vi "AsynCall - MBus Handler.vi"(8 "error in (no error)":errorcluster) -> (0 "error out":errorcluster)   [LabVIEW 2018]
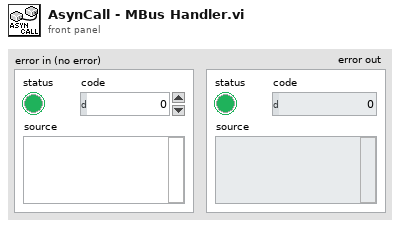
[diagram p1: front panel]
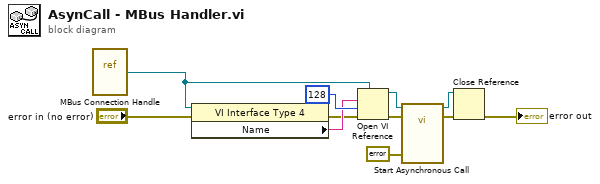
[diagram p0: block diagram]
diagram:
  n1 = vi-ref "MBus Connection Handle.vi"() -> (w3:refnum<vi>)
  n2 = property class="VI Interface Type 4"(reference=w3, error in="error in (no error)") -> (error out=w6:errorcluster, "Name"=w7:string)  [unwired: 1 out]
  n3 = Open VI Reference(type specifier VI Refnum (for type only)=w3, vi path=w7, options=128, error in (no error)=w6) -> (vi reference=w2:refnum<vi>, error out=w8:errorcluster)  [unwired: 2 in]
  n4 = call-by-ref "Start Asynchronous Call"(reference=w2, error in=w8, 8:"error in (no error)"=errorcluster {"status"=FALSE, "code"=0, "source"=""} ("error in (no error)")) -> (reference out=w10:refnum<vi>, error out=w9:errorcluster)  [unwired: 10 in, 1 out]
  n5 = Close Reference(reference=w10, error in (no error)=w9) -> (error out=→"error out":errorcluster)
